vi "Actuator selector.vi"(8 "error in (no error)":errorcluster, 11 "RSA in":refnum<class "RSA.lvclass">) -> (0 "error out":errorcluster, 3 "RSA out":refnum<class "RSA.lvclass">)   [LabVIEW 2012, in "RSA.lvclass"]
uses:
  RSA.lvclass
  RSA.lvclass/RSA.ctl
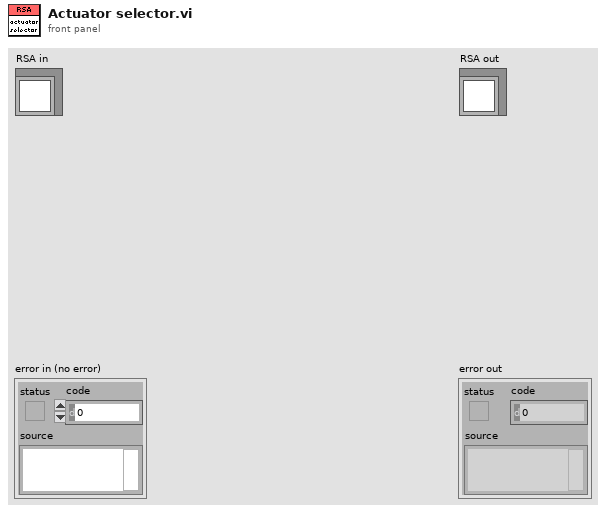
[diagram p1: front panel]
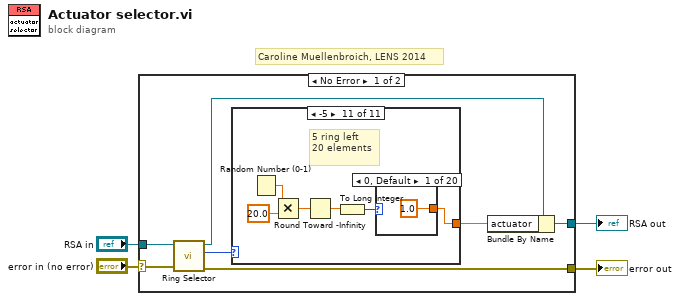
[diagram p0: block diagram]
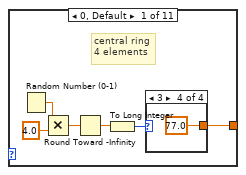
[diagram p2: hidden frame]
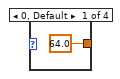
[diagram p3: hidden frame]
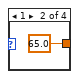
[diagram p4: hidden frame]
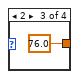
[diagram p5: hidden frame]
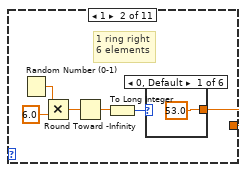
[diagram p6: hidden frame]
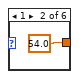
[diagram p7: hidden frame]
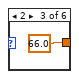
[diagram p8: hidden frame]
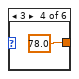
[diagram p9: hidden frame]
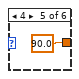
[diagram p10: hidden frame]
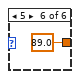
[diagram p11: hidden frame]
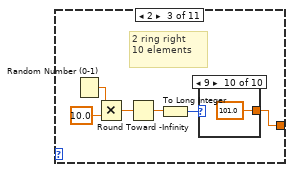
[diagram p12: hidden frame]
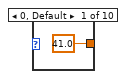
[diagram p13: hidden frame]
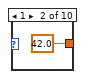
[diagram p14: hidden frame]
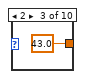
[diagram p15: hidden frame]
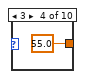
[diagram p16: hidden frame]
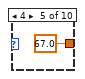
[diagram p17: hidden frame]
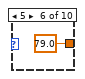
[diagram p18: hidden frame]
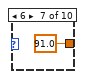
[diagram p19: hidden frame]
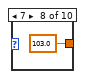
[diagram p20: hidden frame]
diagram:
  # "Caroline Muellenbroich, LENS 2014"
  n1 = case shown="No Error" "error in (no error)" {
    selector: "error in (no error)" -> [w10 w219]
    tunnel: [w8 w219] -> w3
    tunnel: [w6 w218] -> w1
    tunnel: "RSA in" -> [w11 w218]
    frame No Error {
      n2 = call-dynamic "Ring Selector.vi"("error in (no error)"=w10, "RSA in"=w11) -> ("error out"=w8:errorcluster, "Ringnumber"=w9:i32, "RSA out"=w7:refnum<class "RSA.lvclass">)  [unwired: 7 in]
      n3 = case shown="-5" w9 {
        tunnel: [w12 w22 w34 w50 w70 w94 w120 w132 w148 w168 w192] -> w5
        frame 0, Default {
          # "central ring\n4 elements"
          n4 = Random Number (0-1)() -> (number: 0 to 1=w14:dbl)
          n5 = Multiply(x=w14, y=4.0) -> (x*y=w16:dbl)
          n6 = Round Toward -Infinity(1:w16) -> (0:w17:dbl)
          n7 = To Long Integer(number=w17) -> (32bit integer=w13:i32)
          n8 = case shown="3" w13 {
            tunnel: [64.0 ("y") 65.0 ("y") 76.0 ("y") 77.0 ("y")] -> w12
            frame 0, Default {
            }
            frame 1 {
            }
            frame 2 {
            }
            frame 3 {
            }
          }
        }
        frame 1 {
          # "1 ring right\n6 elements"
          n9 = Random Number (0-1)() -> (number: 0 to 1=w26:dbl)
          n10 = Multiply(x=w26, y=6.0) -> (x*y=w24:dbl)
          n11 = Round Toward -Infinity(1:w24) -> (0:w23:dbl)
          n12 = To Long Integer(number=w23) -> (32bit integer=w27:i32)
          n13 = case shown="0, Default" w27 {
            tunnel: [53.0 ("y") 54.0 ("y") 66.0 ("y") 78.0 ("y") 90.0 ("y") 89.0 ("y")] -> w22
            frame 0, Default {
            }
            frame 1 {
            }
            frame 2 {
            }
            frame 3 {
            }
            frame 4 {
            }
            frame 5 {
            }
          }
        }
        frame 2 {
          # "2 ring right\n10 elements"
          n14 = Random Number (0-1)() -> (number: 0 to 1=w38:dbl)
          n15 = Multiply(x=w38, y=10.0) -> (x*y=w36:dbl)
          n16 = Round Toward -Infinity(1:w36) -> (0:w35:dbl)
          n17 = To Long Integer(number=w35) -> (32bit integer=w39:i32)
          n18 = case shown="9" w39 {
            tunnel: [41.0 ("y") 42.0 ("y") 43.0 ("y") 55.0 ("y") 67.0 ("y") 79.0 ("y") 91.0 ("y") 103.0 ("y") 102.0 ("y") 101.0 ("y")] -> w34
            frame 0, Default {
            }
            frame 1 {
            }
            frame 2 {
            }
            frame 3 {
            }
            frame 4 {
            }
            frame 5 {
            }
            frame 6 {
            }
            frame 7 {
            }
            frame 8 {
            }
            frame 9 {
            }
          }
        }
        frame 3 {
          # "3 ring right\n14 elements"
          n19 = Random Number (0-1)() -> (number: 0 to 1=w54:dbl)
          n20 = Multiply(x=w54, y=14.0) -> (x*y=w52:dbl)
          n21 = Round Toward -Infinity(1:w52) -> (0:w51:dbl)
          n22 = To Long Integer(number=w51) -> (32bit integer=w55:i32)
          n23 = case shown="13" w55 {
            tunnel: [29.0 ("y") 30.0 ("y") 31.0 ("y") 32.0 ("y") 44.0 ("y") 56.0 ("y") 68.0 ("y") 80.0 ("y") 92.0 ("y") 104.0 ("y") 116.0 ("y") 115.0 ("y") 114.0 ("y") 113.0 ("y")] -> w50
            frame 0, Default {
            }
            frame 1 {
            }
            frame 2 {
            }
            frame 3 {
            }
            frame 4 {
            }
            frame 5 {
            }
            frame 6 {
            }
            frame 7 {
            }
            frame 8 {
            }
            frame 9 {
            }
            frame 10 {
            }
            frame 11 {
            }
            frame 12 {
            }
            frame 13 {
            }
          }
        }
        frame 4 {
          # "4 ring right\n18 elements"
          n24 = Random Number (0-1)() -> (number: 0 to 1=w74:dbl)
          n25 = Multiply(x=w74, y=18.0) -> (x*y=w72:dbl)
          n26 = Round Toward -Infinity(1:w72) -> (0:w71:dbl)
          n27 = To Long Integer(number=w71) -> (32bit integer=w75:i32)
          n28 = case shown="17" w75 {
            tunnel: [17.0 ("y") 18.0 ("y") 19.0 ("y") 20.0 ("y") 21.0 ("y") 33.0 ("y") 45.0 ("y") 57.0 ("y") 69.0 ("y") 81.0 ("y") 93.0 ("y") 105.0 ("y") 117.0 ("y") 129.0 ("y") 128.0 ("y") 127.0 ("y") 126.0 ("y") 125.0 ("y")] -> w70
            frame 0, Default {
            }
            frame 1 {
            }
            frame 2 {
            }
            frame 3 {
            }
            frame 4 {
            }
            frame 5 {
            }
            frame 6 {
            }
            frame 7 {
            }
            frame 8 {
            }
            frame 9 {
            }
            frame 10 {
            }
            frame 11 {
            }
            frame 12 {
            }
            frame 13 {
            }
            frame 14 {
            }
            frame 15 {
            }
            frame 16 {
            }
            frame 17 {
            }
          }
        }
        frame 5 {
          # "5 ring right\n20 elements"
          n29 = Random Number (0-1)() -> (number: 0 to 1=w98:dbl)
          n30 = Multiply(x=w98, y=20.0) -> (x*y=w96:dbl)
          n31 = Round Toward -Infinity(1:w96) -> (0:w95:dbl)
          n32 = To Long Integer(number=w95) -> (32bit integer=w99:i32)
          n33 = case shown="0, Default" w99 {
            tunnel: [6.0 ("y") 7.0 ("y") 8.0 ("y") 9.0 ("y") 10.0 ("y") 22.0 ("y") 34.0 ("y") 46.0 ("y") 58.0 ("y") 70.0 ("y") 82.0 ("y") 94.0 ("y") 106.0 ("y") 118.0 ("y") 130.0 ("y") 140.0 ("y") 139.0 ("y") 138.0 ("y") 137.0 ("y") 136.0 ("y")] -> w94
            frame 0, Default {
            }
            frame 1 {
            }
            frame 2 {
            }
            frame 3 {
            }
            frame 4 {
            }
            frame 5 {
            }
            frame 6 {
            }
            frame 7 {
            }
            frame 8 {
            }
            frame 9 {
            }
            frame 10 {
            }
            frame 11 {
            }
            frame 12 {
            }
            frame 13 {
            }
            frame 14 {
            }
            frame 15 {
            }
            frame 16 {
            }
            frame 17 {
            }
            frame 18 {
            }
            frame 19 {
            }
          }
        }
        frame -1 {
          # "1 ring left\n6 elements"
          n34 = Random Number (0-1)() -> (number: 0 to 1=w124:dbl)
          n35 = Multiply(x=w124, y=6.0) -> (x*y=w122:dbl)
          n36 = Round Toward -Infinity(1:w122) -> (0:w121:dbl)
          n37 = To Long Integer(number=w121) -> (32bit integer=w125:i32)
          n38 = case shown="0, Default" w125 {
            tunnel: [52.0 ("y") 51.0 ("y") 63.0 ("y") 75.0 ("y") 87.0 ("y") 88.0 ("y")] -> w120
            frame 0, Default {
            }
            frame 1 {
            }
            frame 2 {
            }
            frame 3 {
            }
            frame 4 {
            }
            frame 5 {
            }
          }
        }
        frame -2 {
          # "2 ring left\n10 elements"
          n39 = Random Number (0-1)() -> (number: 0 to 1=w136:dbl)
          n40 = Multiply(x=w136, y=10.0) -> (x*y=w134:dbl)
          n41 = Round Toward -Infinity(1:w134) -> (0:w133:dbl)
          n42 = To Long Integer(number=w133) -> (32bit integer=w137:i32)
          n43 = case shown="0, Default" w137 {
            tunnel: [40.0 ("y") 39.0 ("y") 38.0 ("y") 50.0 ("y") 62.0 ("y") 74.0 ("y") 86.0 ("y") 98.0 ("y") 99.0 ("y") 100.0 ("y")] -> w132
            frame 0, Default {
            }
            frame 1 {
            }
            frame 2 {
            }
            frame 3 {
            }
            frame 4 {
            }
            frame 5 {
            }
            frame 6 {
            }
            frame 7 {
            }
            frame 8 {
            }
            frame 9 {
            }
          }
        }
        frame -3 {
          # "3 ring left\n14 elements"
          n44 = Random Number (0-1)() -> (number: 0 to 1=w152:dbl)
          n45 = Multiply(x=w152, y=14.0) -> (x*y=w150:dbl)
          n46 = Round Toward -Infinity(1:w150) -> (0:w149:dbl)
          n47 = To Long Integer(number=w149) -> (32bit integer=w153:i32)
          n48 = case shown="13" w153 {
            tunnel: [28.0 ("y") 27.0 ("y") 26.0 ("y") 25.0 ("y") 37.0 ("y") 49.0 ("y") 61.0 ("y") 73.0 ("y") 85.0 ("y") 97.0 ("y") 109.0 ("y") 110.0 ("y") 111.0 ("y") 112.0 ("y")] -> w148
            frame 0, Default {
            }
            frame 1 {
            }
            frame 2 {
            }
            frame 3 {
            }
            frame 4 {
            }
            frame 5 {
            }
            frame 6 {
            }
            frame 7 {
            }
            frame 8 {
            }
            frame 9 {
            }
            frame 10 {
            }
            frame 11 {
            }
            frame 12 {
            }
            frame 13 {
            }
          }
        }
        frame -4 {
          # "4 ring left\n18 elements"
          n49 = Random Number (0-1)() -> (number: 0 to 1=w172:dbl)
          n50 = Multiply(x=w172, y=18.0) -> (x*y=w170:dbl)
          n51 = Round Toward -Infinity(1:w170) -> (0:w169:dbl)
          n52 = To Long Integer(number=w169) -> (32bit integer=w173:i32)
          n53 = case shown="17" w173 {
            tunnel: [16.0 ("y") 15.0 ("y") 14.0 ("y") 13.0 ("y") 12.0 ("y") 24.0 ("y") 36.0 ("y") 48.0 ("y") 60.0 ("y") 72.0 ("y") 84.0 ("y") 96.0 ("y") 108.0 ("y") 120.0 ("y") 121.0 ("y") 122.0 ("y") 123.0 ("y") 124.0 ("y")] -> w168
            frame 0, Default {
            }
            frame 1 {
            }
            frame 2 {
            }
            frame 3 {
            }
            frame 4 {
            }
            frame 5 {
            }
            frame 6 {
            }
            frame 7 {
            }
            frame 8 {
            }
            frame 9 {
            }
            frame 10 {
            }
            frame 11 {
            }
            frame 12 {
            }
            frame 13 {
            }
            frame 14 {
            }
            frame 15 {
            }
            frame 16 {
            }
            frame 17 {
            }
          }
        }
        frame -5 {
          # "5 ring left\n20 elements"
          n54 = Random Number (0-1)() -> (number: 0 to 1=w196:dbl)
          n55 = Multiply(x=w196, y=20.0) -> (x*y=w194:dbl)
          n56 = Round Toward -Infinity(1:w194) -> (0:w193:dbl)
          n57 = To Long Integer(number=w193) -> (32bit integer=w197:i32)
          n58 = case shown="0, Default" w197 {
            tunnel: [1.0 ("y") 2.0 ("y") 3.0 ("y") 4.0 ("y") 5.0 ("y") 11.0 ("y") 23.0 ("y") 35.0 ("y") 47.0 ("y") 59.0 ("y") 71.0 ("y") 83.0 ("y") 95.0 ("y") 107.0 ("y") 119.0 ("y") 131.0 ("y") 132.0 ("y") 133.0 ("y") 134.0 ("y") 135.0 ("y")] -> w192
            frame 0, Default {
            }
            frame 1 {
            }
            frame 2 {
            }
            frame 3 {
            }
            frame 4 {
            }
            frame 5 {
            }
            frame 6 {
            }
            frame 7 {
            }
            frame 8 {
            }
            frame 9 {
            }
            frame 10 {
            }
            frame 11 {
            }
            frame 12 {
            }
            frame 13 {
            }
            frame 14 {
            }
            frame 15 {
            }
            frame 16 {
            }
            frame 17 {
            }
            frame 18 {
            }
            frame 19 {
            }
          }
        }
      }
      n59 = Bundle By Name(cluster=w7, "actuator"=w5) -> (w6:refnum<class "RSA.lvclass">)
    }
    frame Error {
    }
  }
  "error out" <- w3
  "RSA out" <- w1
